vi "VIP_Post-Uninstall Custom Action 2021.vi"(10 "Variant":variant) -> (0 "error out":errorcluster)   [LabVIEW 2021]
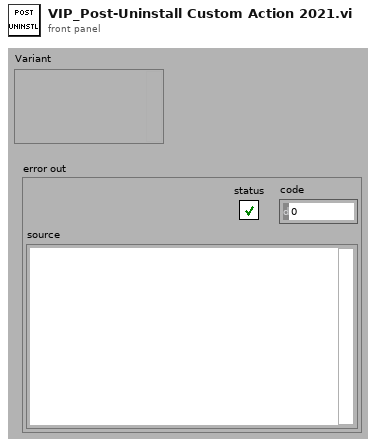
[diagram p1: front panel]
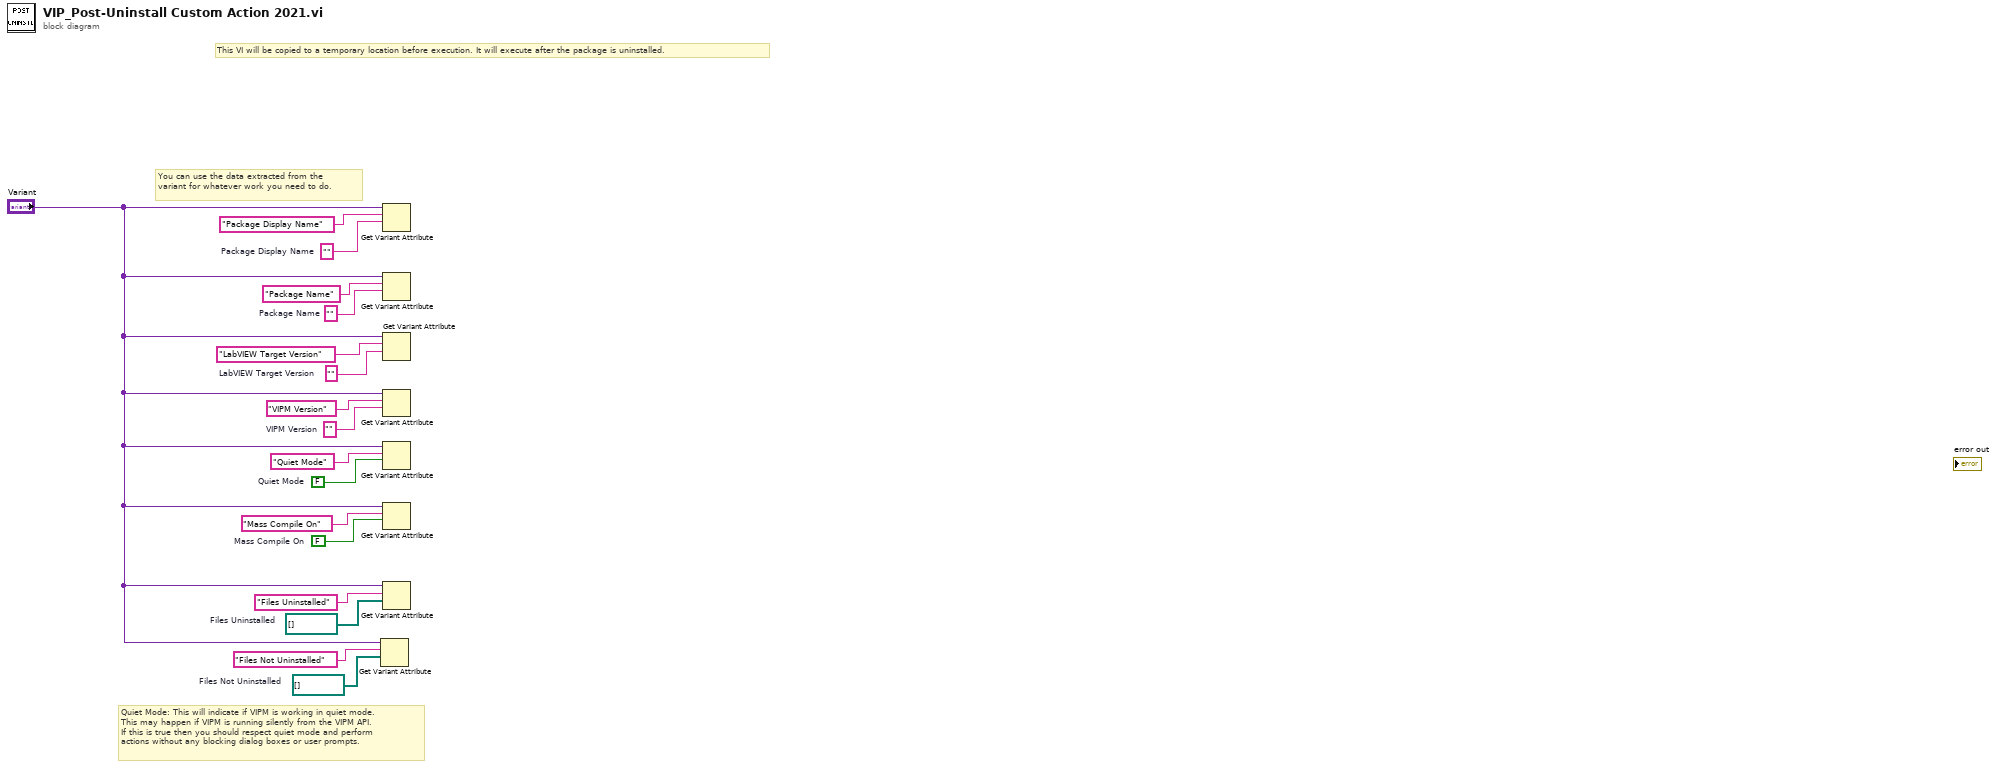
[diagram p0: block diagram]
diagram:
  w1 = path[] []  # Files Not Uninstalled
  w2 = path[] []  # Files Uninstalled
  w6 = FALSE  # Mass Compile On
  w7 = ""  # Package Display Name
  w8 = FALSE  # Quiet Mode
  w11 = ""  # VIPM Version
  w13 = ""  # LabVIEW Target Version
  w15 = ""  # Package Name
  # "You can use the data extracted from the variant for whatever work you need to do."
  # "Quiet Mode: This will indicate if VIPM is working in quiet mode.\nThis may happen if VIPM is running silently from the VIPM API.\nIf this is true then you should respect quiet mode and perform\nactions without any blocking dialog boxes or user prompts."
  # "This VI will be copied to a temporary location before execution. It will execute after the package is uninstalled."
  n1 = Get Variant Attribute(Variant="Variant", name="Files Not Uninstalled", default value (empty Variant)=w1) -> ()  [unwired: 1 in, 4 out]
  n2 = Get Variant Attribute(Variant="Variant", name="Package Display Name", default value (empty Variant)=w7) -> ()  [unwired: 1 in, 4 out]
  n3 = Get Variant Attribute(Variant="Variant", name="Package Name", default value (empty Variant)=w15) -> ()  [unwired: 1 in, 4 out]
  n4 = Get Variant Attribute(Variant="Variant", name="LabVIEW Target Version", default value (empty Variant)=w13) -> ()  [unwired: 1 in, 4 out]
  n5 = Get Variant Attribute(Variant="Variant", name="VIPM Version", default value (empty Variant)=w11) -> ()  [unwired: 1 in, 4 out]
  n6 = Get Variant Attribute(Variant="Variant", name="Quiet Mode", default value (empty Variant)=w8) -> ()  [unwired: 1 in, 4 out]
  n7 = Get Variant Attribute(Variant="Variant", name="Mass Compile On", default value (empty Variant)=w6) -> ()  [unwired: 1 in, 4 out]
  n8 = Get Variant Attribute(Variant="Variant", name="Files Uninstalled", default value (empty Variant)=w2) -> ()  [unwired: 1 in, 4 out]
